vi "WT1800 Configure Instrument.vi"(0 "VISA Refnum in":refnum<visa-resource-name>, 1 "Current Voltage Step":dbl, 2 "Settings Cluster In":T1={"Supply Voltage [Vdc]"=14.4, "Max Supply Current [Idc]"=50.0, "Settling Delay"=0.0, "Temp Criteria"=0.0, "Voltage Steps [Vrms]"=[0.0, 0.25, 0.5, 1.0, 1.95, 3.0, 3.9, 5.5], "User Notes"="", "Config Wave File Path"=path "", "Config Voltage [Vrms]"=0.1, "Channel Configuration List"={"Channel Configuration Cluster"={"Input"=enum."1", "Enable"=FALSE, "User Notes"="", "Voltage Range"=15.0, "Current Range"=2.5}, "Channel Configuration Cluster 2"={"Input"=enum."1", "Enable"=FALSE, "User Notes"="", "Voltage Range"=15.0, "Current Range"=2.5}, "Channel Configuration Cluster 3"={"Input"=enum."1", "Enable"=FALSE, "User Notes"="", "Voltage Range"=15.0, "Current Range"=2.5}, "Channel Configuration Cluster 4"={"Input"=enum."1", "Enable"=FALSE, "User Notes"="", "Voltage Range"=15.0, "Current Range"=2.5}, "Channel Configuration Cluster 5"={"Input"=enum."1", "Enable"=FALSE, "User Notes"="", "Voltage Range"=15.0, "Current Range"=2.5}, "Channel Configuration Cluster 6"={"Input"=enum."1", "Enable"=FALSE, "User Notes"="", "Voltage Range"=15.0, "Current Range"=2.5}, "Channel Configuration Cluster 7"={"Input"=enum."1", "Enable"=FALSE, "User Notes"="", "Voltage Range"=15.0, "Current Range"=2.5}, "Channel Configuration Cluster 8"={"Input"=enum."1", "Enable"=FALSE, "User Notes"="", "Voltage Range"=15.0, "Current Range"=2.5}, "Channel Configuration Cluster 9"={"Input"=enum."1", "Enable"=FALSE, "User Notes"="", "Voltage Range"=15.0, "Current Range"=2.5}, "Channel Configuration Cluster 10"={"Input"=enum."1", "Enable"=FALSE, "User Notes"="", "Voltage Range"=15.0, "Current Range"=25.0}, "Channel Configuration Cluster 11"={"Input"=enum."1", "Enable"=FALSE, "User Notes"="", "Voltage Range"=15.0, "Current Range"=25.0}, "Channel Configuration Cluster 12"={"Input"=enum."1", "Enable"=FALSE, "User Notes"="", "Voltage Range"=15.0, "Current Range"=25.0}, "Channel Configuration Cluster 13"={"Input"=enum."1", "Enable"=FALSE, "User Notes"="", "Voltage Range"=15.0, "Current Range"=25.0}, "Channel Configuration Cluster 14"={"Input"=enum."1", "Enable"=FALSE, "User Notes"="", "Voltage Range"=15.0, "Current Range"=25.0}, "Channel Configuration Cluster 15"={"Input"=enum."1", "Enable"=FALSE, "User Notes"="", "Voltage Range"=15.0, "Current Range"=25.0}, "Channel Configuration Cluster 16"={"Input"=enum."1", "Enable"=FALSE, "User Notes"="", "Voltage Range"=15.0, "Current Range"=25.0}, "Channel Configuration Cluster 17"={"Input"=enum."1", "Enable"=FALSE, "User Notes"="", "Voltage Range"=15.0, "Current Range"=25.0}}, "User Gains"={"Gain 1"=0.0, "Gain 2"=0.0, "Gain 3"=0.0, "Gain 4"=0.0, "Gain 5"=0.0, "Gain 6"=0.0}, "Gains"={"Gain 1"=0.0, "Gain 2"=0.0, "Gain 3"=0.0, "Gain 4"=0.0, "Gain 5"=0.0, "Gain 6"=0.0}, "Gain Array"={"Gain 1"=0.0, "Gain 2"=0.0, "Gain 3"=0.0, "Gain 4"=0.0, "Gain 5"=0.0, "Gain 6"=0.0, "Gain 7"=0.0, "Gain 8"=0.0, "Gain 9"=0.0, "Gain 10"=0.0, "Gain 11"=0.0, "Gain 12"=0.0, "Gain 13"=0.0, "Gain 14"=0.0, "Gain 15"=0.0, "Gain 16"=0.0, "Gain 17"=0.0}, "Wave File Path 1"=path "", "Wave File Path 2"=path "", "Wave File Path 3"=path "", "Wave File Path 4"=path "", "Range"=FALSE, "CF"=FALSE} {"Gain Array"."Gain 17" format="%.2f"; "Gain Array"."Gain 16" format="%.2f"; "Gain Array"."Gain 15" format="%.2f"; "Gain Array"."Gain 14" format="%.2f"; "Gain Array"."Gain 13" format="%.2f"; "Gain Array"."Gain 12" format="%.2f"; "Gain Array"."Gain 11" format="%.2f"; "Gain Array"."Gain 10" format="%.2f"; "Gain Array"."Gain 9" format="%.2f"; "Gain Array"."Gain 8" format="%.2f"; "Gain Array"."Gain 7" format="%.2f"; "Gain Array"."Gain 6" format="%.2f"; "Gain Array"."Gain 5" format="%.2f"; "Gain Array"."Gain 4" format="%.2f"; "Gain Array"."Gain 3" format="%.2f"; "Gain Array"."Gain 2" format="%.2f"; "Gain Array"."Gain 1" format="%.2f"; "Gains"."Gain 6" format="%.2f"; "Gains"."Gain 5" format="%.2f"; "Gains"."Gain 4" format="%.2f"; "Gains"."Gain 3" format="%.2f"; "Gains"."Gain 2" format="%.2f"; "Gains"."Gain 1" format="%.2f"; "User Gains"."Gain 6" format="%.2f"; "User Gains"."Gain 5" format="%.2f"; "User Gains"."Gain 4" format="%.2f"; "User Gains"."Gain 3" format="%.2f"; "User Gains"."Gain 2" format="%.2f"; "User Gains"."Gain 1" format="%.2f"; "Channel Configuration List"."Channel Configuration Cluster 17"."Current Range" items=["1 <500m>"=0.5, "2 <1>"=1.0, "5 <2.5>"=2.5, "10 <5>"=5.0, "20 <10>"=10.0, "50 <25>"=25.0]; "Channel Configuration List"."Channel Configuration Cluster 17"."Voltage Range" items=["1.5 <0.75>"=0.75, "3 <1.5>"=1.5, "6 <3>"=3.0, "10 <5>"=5.0, "15 <7.5>"=7.5, "30 <15>"=15.0, "60 <30>"=30.0, "100 <50>"=50.0, "150 <75>"=75.0, "300 <150>"=150.0, "600 <300>"=300.0, "1000 <500>"=500.0]; "Channel Configuration List"."Channel Configuration Cluster 16"."Current Range" items=["1 <500m>"=0.5, "2 <1>"=1.0, "5 <2.5>"=2.5, "10 <5>"=5.0, "20 <10>"=10.0, "50 <25>"=25.0]; "Channel Configuration List"."Channel Configuration Cluster 16"."Voltage Range" items=["1.5 <0.75>"=0.75, "3 <1.5>"=1.5, "6 <3>"=3.0, "10 <5>"=5.0, "15 <7.5>"=7.5, "30 <15>"=15.0, "60 <30>"=30.0, "100 <50>"=50.0, "150 <75>"=75.0, "300 <150>"=150.0, "600 <300>"=300.0, "1000 <500>"=500.0]; "Channel Configuration List"."Channel Configuration Cluster 15"."Current Range" items=["1 <500m>"=0.5, "2 <1>"=1.0, "5 <2.5>"=2.5, "10 <5>"=5.0, "20 <10>"=10.0, "50 <25>"=25.0]; "Channel Configuration List"."Channel Configuration Cluster 15"."Voltage Range" items=["1.5 <0.75>"=0.75, "3 <1.5>"=1.5, "6 <3>"=3.0, "10 <5>"=5.0, "15 <7.5>"=7.5, "30 <15>"=15.0, "60 <30>"=30.0, "100 <50>"=50.0, "150 <75>"=75.0, "300 <150>"=150.0, "600 <300>"=300.0, "1000 <500>"=500.0]; "Channel Configuration List"."Channel Configuration Cluster 14"."Current Range" items=["1 <500m>"=0.5, "2 <1>"=1.0, "5 <2.5>"=2.5, "10 <5>"=5.0, "20 <10>"=10.0, "50 <25>"=25.0]; "Channel Configuration List"."Channel Configuration Cluster 14"."Voltage Range" items=["1.5 <0.75>"=0.75, "3 <1.5>"=1.5, "6 <3>"=3.0, "10 <5>"=5.0, "15 <7.5>"=7.5, "30 <15>"=15.0, "60 <30>"=30.0, "100 <50>"=50.0, "150 <75>"=75.0, "300 <150>"=150.0, "600 <300>"=300.0, "1000 <500>"=500.0]; "Channel Configuration List"."Channel Configuration Cluster 13"."Current Range" items=["1 <500m>"=0.5, "2 <1>"=1.0, "5 <2.5>"=2.5, "10 <5>"=5.0, "20 <10>"=10.0, "50 <25>"=25.0]; "Channel Configuration List"."Channel Configuration Cluster 13"."Voltage Range" items=["1.5 <0.75>"=0.75, "3 <1.5>"=1.5, "6 <3>"=3.0, "10 <5>"=5.0, "15 <7.5>"=7.5, "30 <15>"=15.0, "60 <30>"=30.0, "100 <50>"=50.0, "150 <75>"=75.0, "300 <150>"=150.0, "600 <300>"=300.0, "1000 <500>"=500.0]; "Channel Configuration List"."Channel Configuration Cluster 12"."Current Range" items=["1 <500m>"=0.5, "2 <1>"=1.0, "5 <2.5>"=2.5, "10 <5>"=5.0, "20 <10>"=10.0, "50 <25>"=25.0]; "Channel Configuration List"."Channel Configuration Cluster 12"."Voltage Range" items=["1.5 <0.75>"=0.75, "3 <1.5>"=1.5, "6 <3>"=3.0, "10 <5>"=5.0, "15 <7.5>"=7.5, "30 <15>"=15.0, "60 <30>"=30.0, "100 <50>"=50.0, "150 <75>"=75.0, "300 <150>"=150.0, "600 <300>"=300.0, "1000 <500>"=500.0]; "Channel Configuration List"."Channel Configuration Cluster 11"."Current Range" items=["1 <500m>"=0.5, "2 <1>"=1.0, "5 <2.5>"=2.5, "10 <5>"=5.0, "20 <10>"=10.0, "50 <25>"=25.0]; "Channel Configuration List"."Channel Configuration Cluster 11"."Voltage Range" items=["1.5 <0.75>"=0.75, "3 <1.5>"=1.5, "6 <3>"=3.0, "10 <5>"=5.0, "15 <7.5>"=7.5, "30 <15>"=15.0, "60 <30>"=30.0, "100 <50>"=50.0, "150 <75>"=75.0, "300 <150>"=150.0, "600 <300>"=300.0, "1000 <500>"=500.0]; "Channel Configuration List"."Channel Configuration Cluster 10"."Current Range" items=["1 <500m>"=0.5, "2 <1>"=1.0, "5 <2.5>"=2.5, "10 <5>"=5.0, "20 <10>"=10.0, "50 <25>"=25.0]; "Channel Configuration List"."Channel Configuration Cluster 10"."Voltage Range" items=["1.5 <0.75>"=0.75, "3 <1.5>"=1.5, "6 <3>"=3.0, "10 <5>"=5.0, "15 <7.5>"=7.5, "30 <15>"=15.0, "60 <30>"=30.0, "100 <50>"=50.0, "150 <75>"=75.0, "300 <150>"=150.0, "600 <300>"=300.0, "1000 <500>"=500.0]; "Channel Configuration List"."Channel Configuration Cluster 9"."Voltage Range" items=["1.5 <0.75>"=0.75, "3 <1.5>"=1.5, "6 <3>"=3.0, "10 <5>"=5.0, "15 <7.5>"=7.5, "30 <15>"=15.0, "60 <30>"=30.0, "100 <50>"=50.0, "150 <75>"=75.0, "300 <150>"=150.0, "600 <300>"=300.0, "1000 <500>"=500.0]; "Channel Configuration List"."Channel Configuration Cluster 9"."Current Range" items=["10m <5m>"=0.005, "20m <10m>"=0.01, "50m <25m>"=0.025, "100m <50m>"=0.05, "200m <100m>"=0.1, "500m <250m>"=0.25, "1 <500m>"=0.5, "2 <1>"=1.0, "5 <2.5>"=2.5]; "Channel Configuration List"."Channel Configuration Cluster 8"."Voltage Range" items=["1.5 <0.75>"=0.75, "3 <1.5>"=1.5, "6 <3>"=3.0, "10 <5>"=5.0, "15 <7.5>"=7.5, "30 <15>"=15.0, "60 <30>"=30.0, "100 <50>"=50.0, "150 <75>"=75.0, "300 <150>"=150.0, "600 <300>"=300.0, "1000 <500>"=500.0]; "Channel Configuration List"."Channel Configuration Cluster 8"."Current Range" items=["10m <5m>"=0.005, "20m <10m>"=0.01, "50m <25m>"=0.025, "100m <50m>"=0.05, "200m <100m>"=0.1, "500m <250m>"=0.25, "1 <500m>"=0.5, "2 <1>"=1.0, "5 <2.5>"=2.5]; "Channel Configuration List"."Channel Configuration Cluster 7"."Voltage Range" items=["1.5 <0.75>"=0.75, "3 <1.5>"=1.5, "6 <3>"=3.0, "10 <5>"=5.0, "15 <7.5>"=7.5, "30 <15>"=15.0, "60 <30>"=30.0, "100 <50>"=50.0, "150 <75>"=75.0, "300 <150>"=150.0, "600 <300>"=300.0, "1000 <500>"=500.0]; "Channel Configuration List"."Channel Configuration Cluster 7"."Current Range" items=["10m <5m>"=0.005, "20m <10m>"=0.01, "50m <25m>"=0.025, "100m <50m>"=0.05, "200m <100m>"=0.1, "500m <250m>"=0.25, "1 <500m>"=0.5, "2 <1>"=1.0, "5 <2.5>"=2.5]; "Channel Configuration List"."Channel Configuration Cluster 6"."Voltage Range" items=["1.5 <0.75>"=0.75, "3 <1.5>"=1.5, "6 <3>"=3.0, "10 <5>"=5.0, "15 <7.5>"=7.5, "30 <15>"=15.0, "60 <30>"=30.0, "100 <50>"=50.0, "150 <75>"=75.0, "300 <150>"=150.0, "600 <300>"=300.0, "1000 <500>"=500.0]; "Channel Configuration List"."Channel Configuration Cluster 6"."Current Range" items=["10m <5m>"=0.005, "20m <10m>"=0.01, "50m <25m>"=0.025, "100m <50m>"=0.05, "200m <100m>"=0.1, "500m <250m>"=0.25, "1 <500m>"=0.5, "2 <1>"=1.0, "5 <2.5>"=2.5]; "Channel Configuration List"."Channel Configuration Cluster 5"."Voltage Range" items=["1.5 <0.75>"=0.75, "3 <1.5>"=1.5, "6 <3>"=3.0, "10 <5>"=5.0, "15 <7.5>"=7.5, "30 <15>"=15.0, "60 <30>"=30.0, "100 <50>"=50.0, "150 <75>"=75.0, "300 <150>"=150.0, "600 <300>"=300.0, "1000 <500>"=500.0]; "Channel Configuration List"."Channel Configuration Cluster 5"."Current Range" items=["10m <5m>"=0.005, "20m <10m>"=0.01, "50m <25m>"=0.025, "100m <50m>"=0.05, "200m <100m>"=0.1, "500m <250m>"=0.25, "1 <500m>"=0.5, "2 <1>"=1.0, "5 <2.5>"=2.5]; "Channel Configuration List"."Channel Configuration Cluster 4"."Voltage Range" items=["1.5 <0.75>"=0.75, "3 <1.5>"=1.5, "6 <3>"=3.0, "10 <5>"=5.0, "15 <7.5>"=7.5, "30 <15>"=15.0, "60 <30>"=30.0, "100 <50>"=50.0, "150 <75>"=75.0, "300 <150>"=150.0, "600 <300>"=300.0, "1000 <500>"=500.0]; "Channel Configuration List"."Channel Configuration Cluster 4"."Current Range" items=["10m <5m>"=0.005, "20m <10m>"=0.01, "50m <25m>"=0.025, "100m <50m>"=0.05, "200m <100m>"=0.1, "500m <250m>"=0.25, "1 <500m>"=0.5, "2 <1>"=1.0, "5 <2.5>"=2.5]; "Channel Configuration List"."Channel Configuration Cluster 3"."Voltage Range" items=["1.5 <0.75>"=0.75, "3 <1.5>"=1.5, "6 <3>"=3.0, "10 <5>"=5.0, "15 <7.5>"=7.5, "30 <15>"=15.0, "60 <30>"=30.0, "100 <50>"=50.0, "150 <75>"=75.0, "300 <150>"=150.0, "600 <300>"=300.0, "1000 <500>"=500.0]; "Channel Configuration List"."Channel Configuration Cluster 3"."Current Range" items=["10m <5m>"=0.005, "20m <10m>"=0.01, "50m <25m>"=0.025, "100m <50m>"=0.05, "200m <100m>"=0.1, "500m <250m>"=0.25, "1 <500m>"=0.5, "2 <1>"=1.0, "5 <2.5>"=2.5]; "Channel Configuration List"."Channel Configuration Cluster 2"."Voltage Range" items=["1.5 <0.75>"=0.75, "3 <1.5>"=1.5, "6 <3>"=3.0, "10 <5>"=5.0, "15 <7.5>"=7.5, "30 <15>"=15.0, "60 <30>"=30.0, "100 <50>"=50.0, "150 <75>"=75.0, "300 <150>"=150.0, "600 <300>"=300.0, "1000 <500>"=500.0]; "Channel Configuration List"."Channel Configuration Cluster 2"."Current Range" items=["10m <5m>"=0.005, "20m <10m>"=0.01, "50m <25m>"=0.025, "100m <50m>"=0.05, "200m <100m>"=0.1, "500m <250m>"=0.25, "1 <500m>"=0.5, "2 <1>"=1.0, "5 <2.5>"=2.5]; "Channel Configuration List"."Channel Configuration Cluster"."Voltage Range" items=["1.5 <0.75>"=0.75, "3 <1.5>"=1.5, "6 <3>"=3.0, "10 <5>"=5.0, "15 <7.5>"=7.5, "30 <15>"=15.0, "60 <30>"=30.0, "100 <50>"=50.0, "150 <75>"=75.0, "300 <150>"=150.0, "600 <300>"=300.0, "1000 <500>"=500.0]; "Channel Configuration List"."Channel Configuration Cluster"."Current Range" items=["10m <5m>"=0.005, "20m <10m>"=0.01, "50m <25m>"=0.025, "100m <50m>"=0.05, "200m <100m>"=0.1, "500m <250m>"=0.25, "1 <500m>"=0.5, "2 <1>"=1.0, "5 <2.5>"=2.5]; "Settling Delay" min=0.0 format="%<%H:%M:%S>t"}, 3 "Channel Config":bool, 5 "Auto Range":bool, 7 "Fixed Range":bool, 9 "Iteration Count":i32, 11 "error in (no error)":errorcluster, 12 "PS Instrument":bool, 13 "Check EQ":bool, 14 "Crest Factor":bool) -> (4 "VISA Refnum out":refnum<visa-resource-name>, 15 "error out":errorcluster)   [LabVIEW 2021]
uses:
  Controls/Settings Control.ctl
  Controls/Channel Configuration List.ctl
  Controls/Channel Configuration Cluster.ctl
  Controls/Channel Configuration Cluster High Current.ctl
  Controls/Gain Averages.ctl
  Controls/Gain Array.ctl
  <instrlib>/Yokogawa WT1800 Series/Public/Configure/Configure Range (Voltage).vi
  <instrlib>/Yokogawa WT1800 Series/Public/Configure/Configure Range (Current 5A).vi
  <instrlib>/Yokogawa WT1800 Series/Public/Configure/Configure Range (Current 50A).vi
  <instrlib>/Yokogawa WT1800 Series/Yokogawa WT1800 Series.lvlib
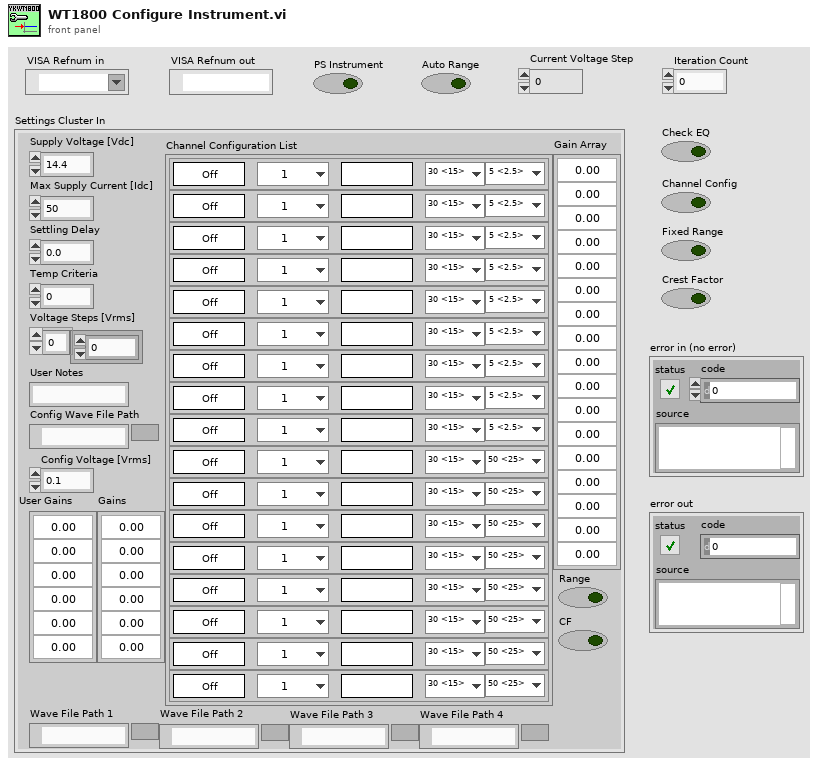
[diagram p1: front panel]
types:
  T1 = typedef "Settings Control.ctl" = cluster{"Supply Voltage [Vdc]":sgl, "Max Supply Current [Idc]":sgl, "Settling Delay":dbl, "Temp Criteria":sgl, "Voltage Steps [Vrms]":sgl[], "User Notes":string, "Config Wave File Path":path, "Config Voltage [Vrms]":sgl, "Channel Configuration List":T2, "User Gains":T5, "Gains":T5, "Gain Array":T6, "Wave File Path 1":path, "Wave File Path 2":path, "Wave File Path 3":path, "Wave File Path 4":path, "Range":bool, "CF":bool}
  T2 = typedef "Channel Configuration List.ctl" = cluster{"Channel Configuration Cluster":T3, "Channel Configuration Cluster 2":T3, "Channel Configuration Cluster 3":T3, "Channel Configuration Cluster 4":T3, "Channel Configuration Cluster 5":T3, "Channel Configuration Cluster 6":T3, "Channel Configuration Cluster 7":T3, "Channel Configuration Cluster 8":T3, "Channel Configuration Cluster 9":T3, "Channel Configuration Cluster 10":T4, "Channel Configuration Cluster 11":T4, "Channel Configuration Cluster 12":T4, "Channel Configuration Cluster 13":T4, "Channel Configuration Cluster 14":T4, "Channel Configuration Cluster 15":T4, "Channel Configuration Cluster 16":T4, "Channel Configuration Cluster 17":T4}
  T3 = typedef "Channel Configuration Cluster.ctl" = cluster{"Input":enum16{"---", "1", "1 AVG", "2", "2 AVG", "3", "3 AVG", "4", "4 AVG"}, "Enable":bool, "User Notes":string, "Voltage Range":dbl, "Current Range":dbl}
  T4 = typedef "Channel Configuration Cluster High Current.ctl" = cluster{"Input":enum16{"---", "1", "1 AVG", "2", "2 AVG", "3", "3 AVG", "4", "4 AVG"}, "Enable":bool, "User Notes":string, "Voltage Range":dbl, "Current Range":dbl}
  T5 = typedef "Gain Averages.ctl" = cluster{"Gain 1":dbl, "Gain 2":dbl, "Gain 3":dbl, "Gain 4":dbl, "Gain 5":dbl, "Gain 6":dbl}
  T6 = typedef "Gain Array.ctl" = cluster{"Gain 1":dbl, "Gain 2":dbl, "Gain 3":dbl, "Gain 4":dbl, "Gain 5":dbl, "Gain 6":dbl, "Gain 7":dbl, "Gain 8":dbl, "Gain 9":dbl, "Gain 10":dbl, "Gain 11":dbl, "Gain 12":dbl, "Gain 13":dbl, "Gain 14":dbl, "Gain 15":dbl, "Gain 16":dbl, "Gain 17":dbl}
  T7 = enum16{"---", "1", "1 AVG", "2", "2 AVG", "3", "3 AVG", "4", "4 AVG"}[]
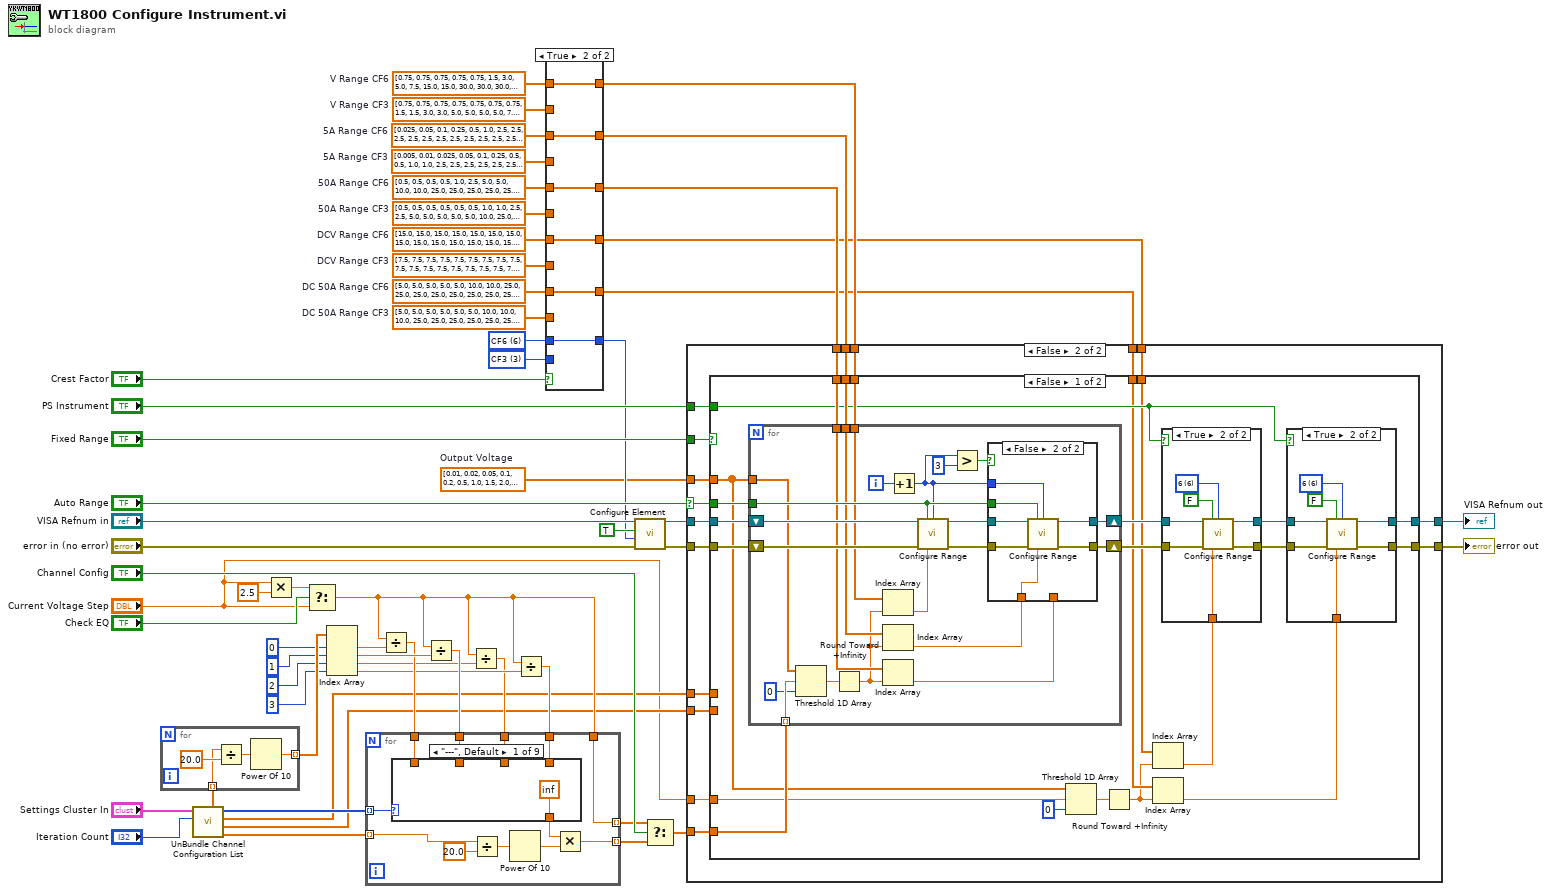
[diagram p0: block diagram]
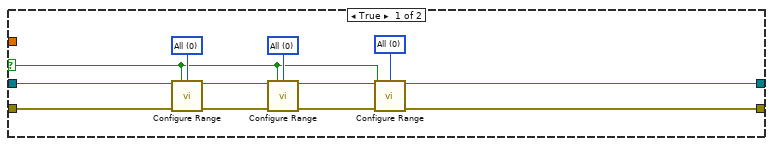
[diagram p11: hidden frame]
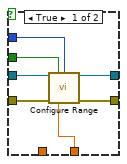
[diagram p14: hidden frame]
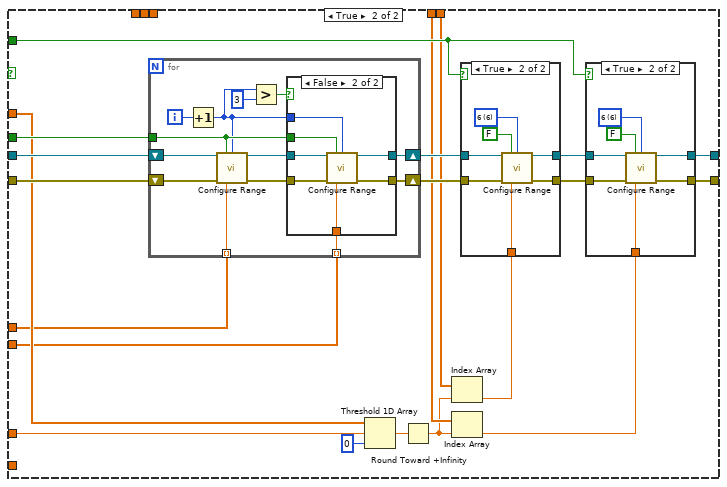
[diagram p15: hidden frame]
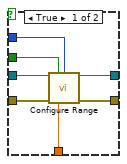
[diagram p18: hidden frame]
diagram:
  w2 = dbl[] [7.5, 7.5, 7.5, 7.5, 7.5, 7.5, 7.5, 7.5, 7.5, 7.5, 7.5, 7.5, 7.5, 7.5, 7.5, 7.5, 7.5, 7.5, 7.5, 7.5, 7.5, 7.5] items=["1.5 <0.75>"=0.75, "3 <1.5>"=1.5, "6 <3>"=3.0, "10 <5>"=5.0, "15 <7.5>"=7.5, "30 <15>"=15.0, "60 <30>"=30.0, "100 <50>"=50.0, "150 <75>"=75.0, "300 <150>"=150.0, "600 <300>"=300.0, "1000 <500>"=500.0]  # DCV Range CF3
  w1 = dbl[] [5.0, 5.0, 5.0, 5.0, 5.0, 5.0, 10.0, 10.0, 10.0, 25.0, 25.0, 25.0, 25.0, 25.0, 25.0, 25.0, 25.0, 25.0, 25.0, 25.0, 25.0, 25.0] items=["1 <500m>"=0.5, "2 <1>"=1.0, "5 <2.5>"=2.5, "10 <5>"=5.0, "20 <10>"=10.0, "50 <25>"=25.0]  # DC 50A Range CF3
  w4 = dbl[] [0.01, 0.02, 0.05, 0.1, 0.2, 0.5, 1.0, 1.5, 2.0, 3.0, 5.0, 6.0, 7.0, 8.0, 9.0, 13.0, 27.0, 50.0, 75.0, 125.0, 270.0, 500.0]  # Output Voltage
  w14 = dbl[] [15.0, 15.0, 15.0, 15.0, 15.0, 15.0, 15.0, 15.0, 15.0, 15.0, 15.0, 15.0, 15.0, 15.0, 15.0, 15.0, 15.0, 15.0, 15.0, 15.0, 15.0, 15.0] items=["1.5 <0.75>"=0.75, "3 <1.5>"=1.5, "6 <3>"=3.0, "10 <5>"=5.0, "15 <7.5>"=7.5, "30 <15>"=15.0, "60 <30>"=30.0, "100 <50>"=50.0, "150 <75>"=75.0, "300 <150>"=150.0, "600 <300>"=300.0, "1000 <500>"=500.0]  # DCV Range CF6
  w13 = dbl[] [5.0, 5.0, 5.0, 5.0, 5.0, 10.0, 10.0, 25.0, 25.0, 25.0, 25.0, 25.0, 25.0, 25.0, 25.0, 25.0, 25.0, 25.0, 25.0, 25.0, 25.0, 25.0] items=["1 <500m>"=0.5, "2 <1>"=1.0, "5 <2.5>"=2.5, "10 <5>"=5.0, "20 <10>"=10.0, "50 <25>"=25.0]  # DC 50A Range CF6
  w12 = dbl[] [0.75, 0.75, 0.75, 0.75, 0.75, 0.75, 0.75, 1.5, 1.5, 3.0, 3.0, 5.0, 5.0, 5.0, 5.0, 7.5, 15.0, 30.0, 50.0, 75.0, 150.0, 300.0] items=["1.5 <0.75>"=0.75, "3 <1.5>"=1.5, "6 <3>"=3.0, "10 <5>"=5.0, "15 <7.5>"=7.5, "30 <15>"=15.0, "60 <30>"=30.0, "100 <50>"=50.0, "150 <75>"=75.0, "300 <150>"=150.0, "600 <300>"=300.0, "1000 <500>"=500.0]  # V Range CF3
  w10 = dbl[] [0.5, 0.5, 0.5, 0.5, 0.5, 0.5, 1.0, 1.0, 2.5, 2.5, 5.0, 5.0, 5.0, 5.0, 5.0, 10.0, 25.0, 25.0, 25.0, 25.0, 25.0, 25.0] items=["1 <500m>"=0.5, "2 <1>"=1.0, "5 <2.5>"=2.5, "10 <5>"=5.0, "20 <10>"=10.0, "50 <25>"=25.0]  # 50A Range CF3
  w16 = dbl[] [0.025, 0.05, 0.1, 0.25, 0.5, 1.0, 2.5, 2.5, 2.5, 2.5, 2.5, 2.5, 2.5, 2.5, 2.5, 2.5, 2.5, 2.5, 2.5, 2.5, 2.5, 2.5] items=["10m <5m>"=0.005, "20m <10m>"=0.01, "50m <25m>"=0.025, "100m <50m>"=0.05, "200m <100m>"=0.1, "500m <250m>"=0.25, "1 <500m>"=0.5, "2 <1>"=1.0, "5 <2.5>"=2.5]  # 5A Range CF6
  w17 = dbl[] [0.75, 0.75, 0.75, 0.75, 0.75, 1.5, 3.0, 5.0, 7.5, 15.0, 15.0, 30.0, 30.0, 30.0, 75.0, 75.0, 75.0, 150.0, 300.0, 500.0, 500.0, 500.0] items=["1.5 <0.75>"=0.75, "3 <1.5>"=1.5, "6 <3>"=3.0, "10 <5>"=5.0, "15 <7.5>"=7.5, "30 <15>"=15.0, "60 <30>"=30.0, "100 <50>"=50.0, "150 <75>"=75.0, "300 <150>"=150.0, "600 <300>"=300.0, "1000 <500>"=500.0]  # V Range CF6
  w15 = dbl[] [0.5, 0.5, 0.5, 0.5, 1.0, 2.5, 5.0, 5.0, 10.0, 10.0, 25.0, 25.0, 25.0, 25.0, 25.0, 25.0, 25.0, 25.0, 25.0, 25.0, 25.0, 25.0] items=["1 <500m>"=0.5, "2 <1>"=1.0, "5 <2.5>"=2.5, "10 <5>"=5.0, "20 <10>"=10.0, "50 <25>"=25.0]  # 50A Range CF6
  w11 = dbl[] [0.005, 0.01, 0.025, 0.05, 0.1, 0.25, 0.5, 0.5, 1.0, 1.0, 2.5, 2.5, 2.5, 2.5, 2.5, 2.5, 2.5, 2.5, 2.5, 2.5, 2.5, 2.5] items=["10m <5m>"=0.005, "20m <10m>"=0.01, "50m <25m>"=0.025, "100m <50m>"=0.05, "200m <100m>"=0.1, "500m <250m>"=0.25, "1 <500m>"=0.5, "2 <1>"=1.0, "5 <2.5>"=2.5]  # 5A Range CF3
  w18 = 3 items=["CF3"=3, "CF6"=6] ("Crest Factor (3: CF3)")
  w20 = 6 items=["CF3"=3, "CF6"=6] ("Crest Factor (3: CF3)")
  n1 = call "UnBundle Channel Configuration List.vi"("Iteration Count"="Iteration Count", "Settings Cluster In"="Settings Cluster In") -> ("Gain Array"=w31:dbl[], "Current Range"=w22:dbl[], "Voltage Range"=w23:dbl[], "Input"=w29:T7, "User Gains"=w30:dbl[])  [unwired: 5 in]
  n2 = for {
    tunnel: w30 -> [w61] mode=indexing
    tunnel: [w60] -> w54 mode=indexing
    n3 = Divide(x=w61, y=20.0) -> (x/y=w62:dbl)
    n4 = Power Of 10(x=w62) -> (10^x=w60:dbl)
  }
  n5 = Multiply(x="Current Voltage Step", y=2.5) -> (x*y=w40:dbl)
  n6 = Select(t=w40, s="Check EQ", f="Current Voltage Step") -> (s? t:f=w36:dbl)
  n7 = Index Array(array=w54, index #1=0 ("index"), index #2=1 ("index"), index #3=2 ("index"), index #4=3 ("index")) -> (element #1=w51:dbl, element #2=w50:dbl, element #3=w35:dbl, element #4=w34:dbl)
  n8 = Divide(x=w36, y=w51) -> (x/y=w48:dbl)
  n9 = Divide(x=w36, y=w50) -> (x/y=w49:dbl)
  n10 = Divide(x=w36, y=w35) -> (x/y=w33:dbl)
  n11 = Divide(x=w36, y=w34) -> (x/y=w32:dbl)
  n12 = for {
    tunnel: w31 -> [w72] mode=indexing
    tunnel: w49 -> [w69]
    tunnel: w48 -> [w70]
    tunnel: [w68] -> w47 mode=indexing
    tunnel: [w67] -> w44 mode=indexing
    tunnel: w36 -> [w67]
    tunnel: w33 -> [w66]
    tunnel: w32 -> [w65]
    tunnel: w29 -> [w64] mode=indexing
    n13 = case shown="\"---\", Default" w64 {
      tunnel: [inf w77 w78 w79 w80 w81 w82 w83 w84] -> w71
      tunnel: w70 -> [_ w77 w78 _ _ _ _ _ _]
      tunnel: w69 -> [_ _ _ w79 w80 _ _ _ _]
      tunnel: w66 -> [_ _ _ _ _ w81 w82 _ _]
      tunnel: w65 -> [_ _ _ _ _ _ _ w83 w84]
      frame "---", Default {
      }
      frame "1" {
      }
      frame "1 AVG" {
      }
      frame "2" {
      }
      frame "2 AVG" {
      }
      frame "3" {
      }
      frame "3 AVG" {
      }
      frame "4" {
      }
      frame "4 AVG" {
      }
    }
    n14 = Divide(x=w72, y=20.0) -> (x/y=w75:dbl)
    n15 = Power Of 10(x=w75) -> (10^x=w73:dbl)
    n16 = Multiply(x=w71, y=w73) -> (x*y=w68:dbl)
  }
  n17 = case shown="True" "Crest Factor" {
    tunnel: [w90 w96] -> w19
    tunnel: w20 -> [_ w96]
    tunnel: w18 -> [w90 _]
    tunnel: [w89 w95] -> w9
    tunnel: w17 -> [_ w95]
    tunnel: [w88 w94] -> w8
    tunnel: w16 -> [_ w94]
    tunnel: [w87 w93] -> w7
    tunnel: w15 -> [_ w93]
    tunnel: [w86 w92] -> w6
    tunnel: w14 -> [_ w92]
    tunnel: [w85 w91] -> w5
    tunnel: w13 -> [_ w91]
    tunnel: w12 -> [w89 _]
    tunnel: w11 -> [w88 _]
    tunnel: w10 -> [w87 _]
    tunnel: w2 -> [w86 _]
    tunnel: w1 -> [w85 _]
    frame False {
    }
    frame True {
    }
  }
  n18 = call <instrlib>:"Configure Element.vi"("error in (no error)"="error in (no error)", "Crest Factor (3: CF3)"=w19, "Enable Independent Element (F: Disable)"=TRUE, "VISA resource name"="VISA Refnum in") -> ("error out"=w27:errorcluster, "VISA resource name out"=w25:refnum<visa-resource-name>)  [unwired: 6 in]
  n19 = Select(t=w44, s="Channel Config", f=w47) -> (s? t:f=w46:dbl[])
  n20 = case shown="False" "Auto Range" {
    selector: "Auto Range" -> [w97 w125]
    tunnel: w27 -> [w105 w124]
    tunnel: [w99 w122] -> w57
    tunnel: w25 -> [w106 w123]
    tunnel: [w101 w121] -> w58
    tunnel: "PS Instrument" -> [_ w120]
    tunnel: w46 -> [_ w119]
    tunnel: "Fixed Range" -> [_ w118]
    tunnel: w23 -> [_ w117]
    tunnel: w22 -> [_ w116]
    tunnel: w9 -> [_ w115]
    tunnel: w8 -> [_ w114]
    tunnel: w7 -> [_ w113]
    tunnel: w6 -> [_ w112]
    tunnel: w5 -> [_ w111]
    tunnel: w4 -> [_ w110]
    tunnel: "Current Voltage Step" -> [_ w109]
    frame True {
      w98 = 0 items=["All", "1", "2", "3", "4", "5", "6"] ("Element (0:All)")
      w103 = 0 items=["All", "1", "2", "3", "4", "5", "6"] ("Element (0:All)")
      w104 = 0 items=["All", "1", "2", "3", "4", "5", "6"] ("Element (0:All)")
      n21 = call-poly <instrlib>:"Configure Range.vi"("VISA resource name"=w106, "Auto Range (F: Disable)"=w97, "Element (0:All)"=w103, "error in (no error)"=w105) -> ("VISA resource name out"=w107:refnum<visa-resource-name>, "error out"=w108:errorcluster)  [unwired: 10 in]
      n22 = call-poly <instrlib>:"Configure Range.vi"("VISA resource name"=w107, "Auto Range (F: Disable)"=w97, "Element (0:All)"=w104, "error in (no error)"=w108) -> ("VISA resource name out"=w102:refnum<visa-resource-name>, "error out"=w100:errorcluster)  [unwired: 10 in]
      n23 = call-poly <instrlib>:"Configure Range.vi"("VISA resource name"=w102, "Auto Range (F: Disable)"=w97, "Element (0:All)"=w98, "error in (no error)"=w100) -> ("VISA resource name out"=w101:refnum<visa-resource-name>, "error out"=w99:errorcluster)  [unwired: 10 in]
    }
    frame False {
      n24 = case shown="False" w118 {
        tunnel: w125 -> [w148 w223]
        tunnel: w124 -> [w147 w222]
        tunnel: w123 -> [w146 w221]
        tunnel: [w136 w215] -> w122
        tunnel: [w137 w216] -> w121
        tunnel: w120 -> [w139 w218]
        tunnel: w119 -> [w145 _]
        tunnel: w117 -> [_ w204]
        tunnel: w116 -> [_ w203]
        tunnel: w115 -> [w144 _]
        tunnel: w114 -> [w143 _]
        tunnel: w113 -> [w142 _]
        tunnel: w112 -> [w132 w211]
        tunnel: w111 -> [w134 w213]
        tunnel: w110 -> [w126 w205]
        tunnel: w109 -> [w127 w206]
        frame False {
          n25 = for {
            tunnel: w148 -> [w188]
            tunnel: w145 -> [w185] mode=indexing
            shift-right: [w168] -> w135
            shift-left: w147 -> [w187]
            shift-right: [w169] -> w138
            shift-left: w146 -> [w186]
            tunnel: w144 -> [w173]
            tunnel: w143 -> [w172]
            tunnel: w142 -> [w171]
            tunnel: w126 -> [w170]
            i -> [w178]
            n26 = Threshold 1D Array(1:0 ("start index (0)"), 2:w185, 3:w170) -> (0:w184:dbl)
            n27 = Round Toward +Infinity(x=w184) -> (ceil(x): smallest int >= x=w167:dbl)
            n28 = Index Array(array=w173, index=w167) -> (element=w183:dbl)
            n29 = Index Array(array=w172, index=w167) -> (element=w182:dbl)
            n30 = Index Array(array=w171, index=w167) -> (element=w174:dbl)
            n31 = Increment(x=w178) -> (x+1=w177:i32)
            n32 = call-poly <instrlib>:"Configure Range.vi"("VISA resource name"=w186, "Auto Range (F: Disable)"=w188, "Element (0:All)"=w177, "error in (no error)"=w187, "Manual Range (1000 <500> V)"=w183) -> ("VISA resource name out"=w181:refnum<visa-resource-name>, "error out"=w180:errorcluster)  [unwired: 9 in]
            n33 = Greater?(x=w177, y=3) -> (0:w175:bool)
            n34 = case shown="False" w175 {
              tunnel: w188 -> [w195 w202]
              tunnel: [w194 w201] -> w169
              tunnel: [w193 w200] -> w168
              tunnel: w182 -> [_ w196]
              tunnel: w181 -> [w192 w199]
              tunnel: w180 -> [w191 w198]
              tunnel: w177 -> [w190 w197]
              tunnel: w174 -> [w189 _]
              frame True {
                n35 = call-poly <instrlib>:"Configure Range.vi"("VISA resource name"=w192, "Auto Range (F: Disable)"=w195, "Element (0:All)"=w190, "error in (no error)"=w191, "Manual Range (50 <25> A)"=w189) -> ("VISA resource name out"=w194:refnum<visa-resource-name>, "error out"=w193:errorcluster)  [unwired: 9 in]
              }
              frame False {
                n36 = call-poly <instrlib>:"Configure Range.vi"("VISA resource name"=w199, "Auto Range (F: Disable)"=w202, "Element (0:All)"=w197, "error in (no error)"=w198, "Manual Range (5 <2.5> A)"=w196) -> ("VISA resource name out"=w201:refnum<visa-resource-name>, "error out"=w200:errorcluster)  [unwired: 9 in]
              }
            }
          }
          n37 = Threshold 1D Array(1:0 ("start index (0)"), 2:w127, 3:w126) -> (0:w130:dbl)
          n38 = Round Toward +Infinity(x=w130) -> (ceil(x): smallest int >= x=w128:dbl)
          n39 = Index Array(array=w132, index=w128) -> (element=w131:dbl)
          n40 = Index Array(array=w134, index=w128) -> (element=w133:dbl)
          n41 = case shown="True" w139 {
            tunnel: w138 -> [w150 w155]
            tunnel: [w150 w154] -> w140
            tunnel: w135 -> [w149 w153]
            tunnel: [w149 w152] -> w141
            tunnel: w131 -> [_ w151]
            frame False {
            }
            frame True {
              w156 = 6 items=["All", "1", "2", "3", "4", "5", "6"] ("Element (0:All)")
              n42 = call-poly <instrlib>:"Configure Range.vi"("VISA resource name"=w155, "Auto Range (F: Disable)"=FALSE, "Element (0:All)"=w156, "error in (no error)"=w153, "Manual Range (1000 <500> V)"=w151) -> ("VISA resource name out"=w154:refnum<visa-resource-name>, "error out"=w152:errorcluster)  [unwired: 9 in]
            }
          }
          n43 = case shown="True" w139 {
            tunnel: w133 -> [_ w164]
            tunnel: w141 -> [w158 w163]
            tunnel: [w158 w162] -> w136
            tunnel: w140 -> [w159 w161]
            tunnel: [w159 w160] -> w137
            frame False {
            }
            frame True {
              w165 = 6 items=["All", "1", "2", "3", "4", "5", "6"] ("Element (0:All)")
              n44 = call-poly <instrlib>:"Configure Range.vi"("VISA resource name"=w161, "Auto Range (F: Disable)"=FALSE, "Element (0:All)"=w165, "error in (no error)"=w163, "Manual Range (50 <25> A)"=w164) -> ("VISA resource name out"=w160:refnum<visa-resource-name>, "error out"=w162:errorcluster)  [unwired: 9 in]
            }
          }
        }
        frame True {
          n45 = for {
            tunnel: w223 -> [w254]
            shift-right: [w244] -> w214
            shift-left: w222 -> [w253]
            shift-right: [w245] -> w217
            shift-left: w221 -> [w252]
            tunnel: w204 -> [w243] mode=indexing
            tunnel: w203 -> [w242] mode=indexing
            i -> [w249]
            n46 = Increment(x=w249) -> (x+1=w248:i32)
            n47 = call-poly <instrlib>:"Configure Range.vi"("VISA resource name"=w252, "Auto Range (F: Disable)"=w254, "Element (0:All)"=w248, "error in (no error)"=w253, "Manual Range (1000 <500> V)"=w243) -> ("VISA resource name out"=w251:refnum<visa-resource-name>, "error out"=w250:errorcluster)  [unwired: 9 in]
            n48 = Greater?(x=w248, y=3) -> (0:w246:bool)
            n49 = case shown="False" w246 {
              tunnel: w254 -> [w261 w268]
              tunnel: [w260 w267] -> w245
              tunnel: [w259 w266] -> w244
              tunnel: w242 -> [w255 w262]
              tunnel: w251 -> [w258 w265]
              tunnel: w250 -> [w257 w264]
              tunnel: w248 -> [w256 w263]
              frame True {
                n50 = call-poly <instrlib>:"Configure Range.vi"("VISA resource name"=w258, "Auto Range (F: Disable)"=w261, "Element (0:All)"=w256, "error in (no error)"=w257, "Manual Range (50 <25> A)"=w255) -> ("VISA resource name out"=w260:refnum<visa-resource-name>, "error out"=w259:errorcluster)  [unwired: 9 in]
              }
              frame False {
                n51 = call-poly <instrlib>:"Configure Range.vi"("VISA resource name"=w265, "Auto Range (F: Disable)"=w268, "Element (0:All)"=w263, "error in (no error)"=w264, "Manual Range (5 <2.5> A)"=w262) -> ("VISA resource name out"=w267:refnum<visa-resource-name>, "error out"=w266:errorcluster)  [unwired: 9 in]
              }
            }
          }
          n52 = Threshold 1D Array(1:0 ("start index (0)"), 2:w206, 3:w205) -> (0:w209:dbl)
          n53 = Round Toward +Infinity(x=w209) -> (ceil(x): smallest int >= x=w207:dbl)
          n54 = Index Array(array=w211, index=w207) -> (element=w210:dbl)
          n55 = Index Array(array=w213, index=w207) -> (element=w212:dbl)
          n56 = case shown="True" w218 {
            tunnel: w217 -> [w225 w230]
            tunnel: [w225 w229] -> w219
            tunnel: w214 -> [w224 w228]
            tunnel: [w224 w227] -> w220
            tunnel: w210 -> [_ w226]
            frame False {
            }
            frame True {
              w231 = 6 items=["All", "1", "2", "3", "4", "5", "6"] ("Element (0:All)")
              n57 = call-poly <instrlib>:"Configure Range.vi"("VISA resource name"=w230, "Auto Range (F: Disable)"=FALSE, "Element (0:All)"=w231, "error in (no error)"=w228, "Manual Range (1000 <500> V)"=w226) -> ("VISA resource name out"=w229:refnum<visa-resource-name>, "error out"=w227:errorcluster)  [unwired: 9 in]
            }
          }
          n58 = case shown="True" w218 {
            tunnel: w212 -> [_ w239]
            tunnel: w220 -> [w233 w238]
            tunnel: [w233 w237] -> w215
            tunnel: w219 -> [w234 w236]
            tunnel: [w234 w235] -> w216
            frame False {
            }
            frame True {
              w240 = 6 items=["All", "1", "2", "3", "4", "5", "6"] ("Element (0:All)")
              n59 = call-poly <instrlib>:"Configure Range.vi"("VISA resource name"=w236, "Auto Range (F: Disable)"=FALSE, "Element (0:All)"=w240, "error in (no error)"=w238, "Manual Range (50 <25> A)"=w239) -> ("VISA resource name out"=w235:refnum<visa-resource-name>, "error out"=w237:errorcluster)  [unwired: 9 in]
            }
          }
        }
      }
    }
  }
  "VISA Refnum out" <- w58
  "error out" <- w57
